vi "AppendFrontPanelImageToReport_Mutation.vi"(0 "Diagram":refnum<vi>, 5 "ObjRef":refnum<vi>, 6 "Kind":string="SubVI", 7 "Information":string="<Not A Path>") -> (3 "Replace?":bool)   [LabVIEW 2020]
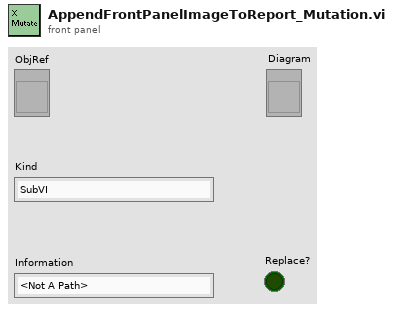
[diagram p1: front panel]
types:
  T1 = typedef "LVPositionTypeDef.ctl" = cluster{"Left":i32, "Top":i32}
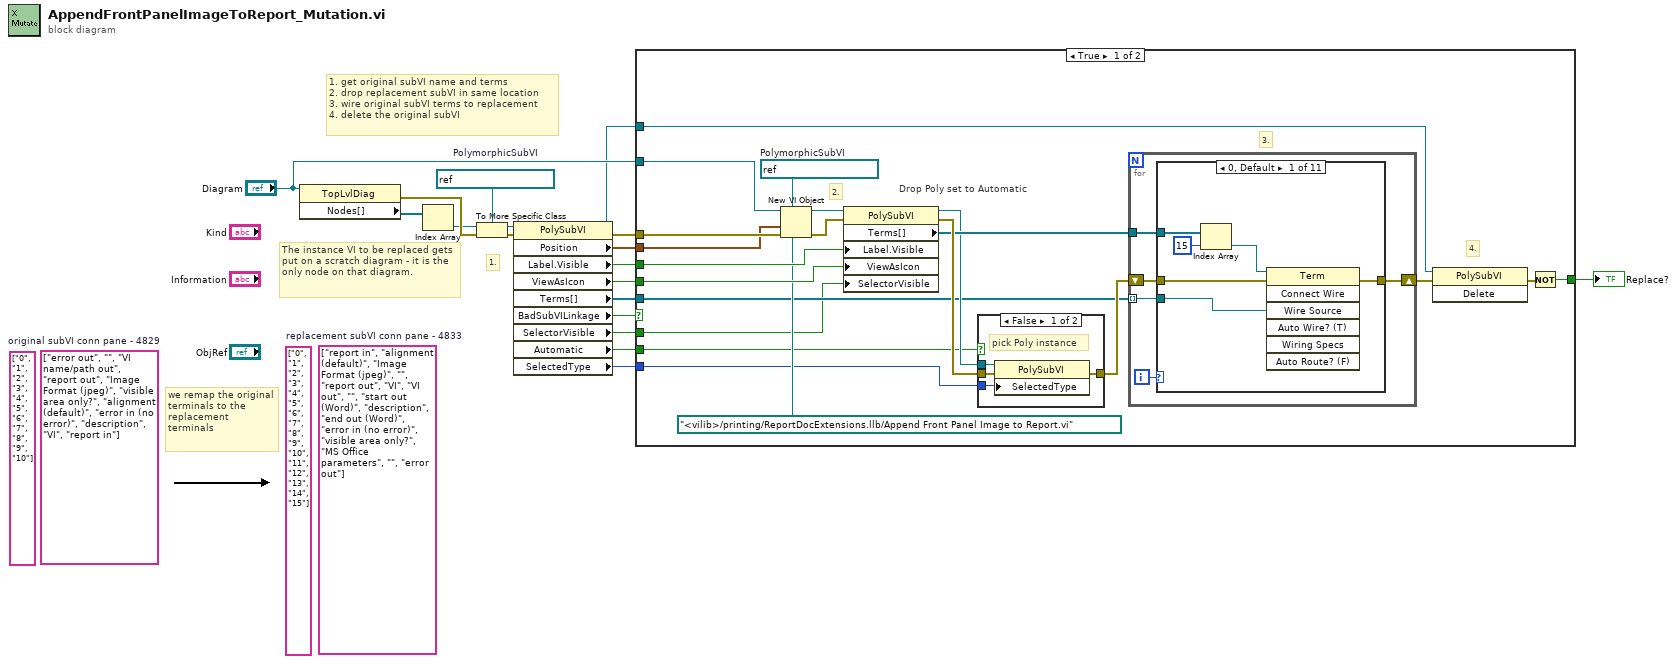
[diagram p0: block diagram]
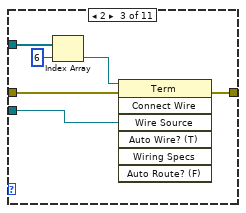
[diagram p4: hidden frame]
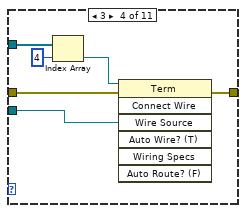
[diagram p5: hidden frame]
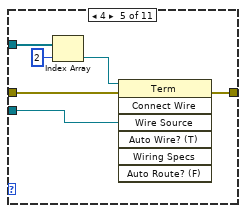
[diagram p6: hidden frame]
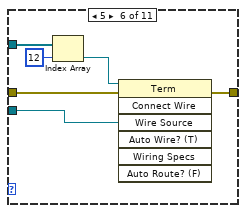
[diagram p7: hidden frame]
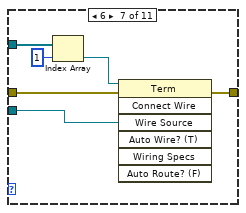
[diagram p8: hidden frame]
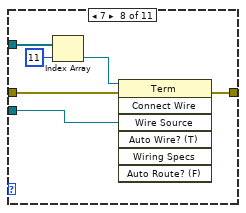
[diagram p9: hidden frame]
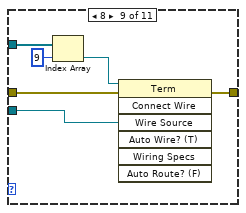
[diagram p10: hidden frame]
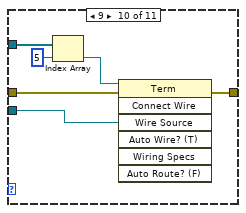
[diagram p11: hidden frame]
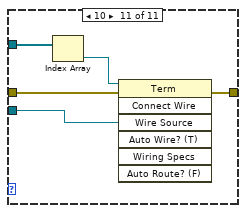
[diagram p12: hidden frame]
diagram:
  w5 = refnum<vi> refnum  # PolymorphicSubVI
  (unwired) string[] ["0", "1", "2", "3", "4", "5", "6", "7", "8", "9", "10", "11", "12", "13", "14", "15"]
  (unwired) string[] ["0", "1", "2", "3", "4", "5", "6", "7", "8", "9", "10"]
  (unwired) string[] ["report in", "alignment (default)", "Image Format (jpeg)", "", "report out", "VI", "VI out", "", "start out (Word)", "description", "end out (Word)", "error in (no error)", "visible area only?", "MS Office parameters", "", "error out"]  # replacement subVI conn pane - 4833
  (unwired) string[] ["error out", "", "VI name/path out", "report out", "Image Format (jpeg)", "visible area only?", "alignment (default)", "error in (no error)", "description", "VI", "report in"]  # original subVI conn pane - 4829
  # "1."
  # "we remap the original terminals to the replacement terminals"
  # "The instance VI to be replaced gets put on a scratch diagram - it is the only node on that diagram."
  # "1. get original subVI name and terms\n2. drop replacement subVI in same location\n3. wire original subVI terms to replacement\n4. delete the original subVI"
  n1 = property class="TopLvlDiag"(reference="Diagram") -> (error out=w17:errorcluster, "Nodes[]"=w15:refnum<vi>[])  [unwired: 1 in, 1 out]
  n2 = Index Array(array=w15) -> (element=w14:refnum<vi>)  [unwired: 1 in]
  n3 = To More Specific Class(target class=w5, reference=w14, error in=w17) -> (specific class reference=w6:refnum<vi>, error out=w18:errorcluster)
  n4 = property class="PolySubVI"(reference=w6, error in=w18) -> (reference out=w9:refnum<vi>, error out=w16:errorcluster, "Position"=w10:T1, "Label.Visible"=w13:bool, "ViewAsIcon"=w12:bool, "Terms[]"=w7:refnum<vi>[], "BadSubVILinkage"=w2:bool, "SelectorVisible"=w1:bool, "Automatic"=w4:bool, "SelectedType"=w3:i32)
  n5 = case shown="True" w2 {
    tunnel: w13 -> [w32 _]
    tunnel: w12 -> [w31 _]
    tunnel: "Diagram" -> [w30 _]
    tunnel: w10 -> [w29 _]
    tunnel: w9 -> [w28 _]
    tunnel: [w27 _] -> w8
    tunnel: w16 -> [w38 _]
    tunnel: w7 -> [w21 _]
    tunnel: w4 -> [w22 _]
    tunnel: w3 -> [w20 _]
    tunnel: w1 -> [w19 _]
    frame True {
      w24 = refnum<vi> refnum  # PolymorphicSubVI
      # "Drop Poly set to Automatic"
      # "4."
      # "3."
      # "2."
      n6 = New VI Object(vi object class=w24, owner refnum=w30, position/next to=w29, 6:path "<vilib>/printing/ReportDocExtensions.llb/Append Front Panel Image to Report.vi", 8:w38) -> (object refnum=w33:refnum<vi>, 0:w37:errorcluster)  [unwired: 3 in]
      n7 = property class="PolySubVI"(reference=w33, error in=w37, "Label.Visible"=w32, "ViewAsIcon"=w31, "SelectorVisible"=w19) -> (reference out=w23:refnum<vi>, error out=w35:errorcluster, "Terms[]"=w26:refnum<vi>[])
      n8 = case shown="False" w22 {
        tunnel: w23 -> [w41 _]
        tunnel: w35 -> [w43 w44]
        tunnel: [w42 w44] -> w34
        tunnel: w20 -> [w40 _]
        frame False {
          # "pick Poly instance"
          n9 = property class="PolySubVI"(reference=w41, error in=w43, "SelectedType"=w40) -> (error out=w42:errorcluster)  [unwired: 1 out]
        }
        frame True {
        }
      }
      n10 = for {
        tunnel: w21 -> [w46] mode=indexing
        tunnel: w26 -> [w45]
        shift-right: [w48] -> w39
        shift-left: w34 -> [w49]
        i -> [w47]
        n11 = case shown="0, Default" w47 {
          tunnel: w46 -> [w53 _ w60 w66 w72 w78 w84 w90 w96 w102 w107]
          tunnel: w45 -> [w52 _ w59 w65 w71 w77 w83 w89 w95 w101 w106]
          tunnel: w49 -> [w55 w56 w62 w68 w74 w80 w86 w92 w98 w104 w109]
          tunnel: [w54 w56 w61 w67 w73 w79 w85 w91 w97 w103 w108] -> w48
          frame 0, Default {
            n12 = Index Array(array=w52, index=15) -> (element=w50:refnum<vi>)
            n13 = invoke class="Term" method="Connect Wire"(reference=w50, error in=w55, "Wire Source"=w53) -> (error out=w54:errorcluster)  [unwired: 4 in, 6 out]
          }
          frame 1 {
          }
          frame 2 {
            n14 = Index Array(array=w59, index=6) -> (element=w57:refnum<vi>)
            n15 = invoke class="Term" method="Connect Wire"(reference=w57, error in=w62, "Wire Source"=w60) -> (error out=w61:errorcluster)  [unwired: 4 in, 6 out]
          }
          frame 3 {
            n16 = Index Array(array=w65, index=4) -> (element=w63:refnum<vi>)
            n17 = invoke class="Term" method="Connect Wire"(reference=w63, error in=w68, "Wire Source"=w66) -> (error out=w67:errorcluster)  [unwired: 4 in, 6 out]
          }
          frame 4 {
            n18 = Index Array(array=w71, index=2) -> (element=w69:refnum<vi>)
            n19 = invoke class="Term" method="Connect Wire"(reference=w69, error in=w74, "Wire Source"=w72) -> (error out=w73:errorcluster)  [unwired: 4 in, 6 out]
          }
          frame 5 {
            n20 = Index Array(array=w77, index=12) -> (element=w75:refnum<vi>)
            n21 = invoke class="Term" method="Connect Wire"(reference=w75, error in=w80, "Wire Source"=w78) -> (error out=w79:errorcluster)  [unwired: 4 in, 6 out]
          }
          frame 6 {
            n22 = Index Array(array=w83, index=1) -> (element=w81:refnum<vi>)
            n23 = invoke class="Term" method="Connect Wire"(reference=w81, error in=w86, "Wire Source"=w84) -> (error out=w85:errorcluster)  [unwired: 4 in, 6 out]
          }
          frame 7 {
            n24 = Index Array(array=w89, index=11) -> (element=w87:refnum<vi>)
            n25 = invoke class="Term" method="Connect Wire"(reference=w87, error in=w92, "Wire Source"=w90) -> (error out=w91:errorcluster)  [unwired: 4 in, 6 out]
          }
          frame 8 {
            n26 = Index Array(array=w95, index=9) -> (element=w93:refnum<vi>)
            n27 = invoke class="Term" method="Connect Wire"(reference=w93, error in=w98, "Wire Source"=w96) -> (error out=w97:errorcluster)  [unwired: 4 in, 6 out]
          }
          frame 9 {
            n28 = Index Array(array=w101, index=5) -> (element=w99:refnum<vi>)
            n29 = invoke class="Term" method="Connect Wire"(reference=w99, error in=w104, "Wire Source"=w102) -> (error out=w103:errorcluster)  [unwired: 4 in, 6 out]
          }
          frame 10 {
            n30 = Index Array(array=w106) -> (element=w105:refnum<vi>)  [unwired: 1 in]
            n31 = invoke class="Term" method="Connect Wire"(reference=w105, error in=w109, "Wire Source"=w107) -> (error out=w108:errorcluster)  [unwired: 4 in, 6 out]
          }
        }
      }
      n32 = invoke class="PolySubVI" method="Delete"(reference=w28, error in=w39) -> (error out=w36:errorcluster)  [unwired: 1 in, 2 out]
      n33 = Not(x=w36) -> (.not. x?=w27:bool)
    }
    frame False {
    }
  }
  "Replace?" <- w8
